vi "UpdateMovingCursor XYGraph.vi"(8 "Coords":T1, 9 "CtlRef":refnum<vi>) -> ()   [LabVIEW 2013, in "main.lvlib"]
uses:
  main.lvlib
  <vilib>/Utility/miscctls.llb/LVPoint32TypeDef.ctl
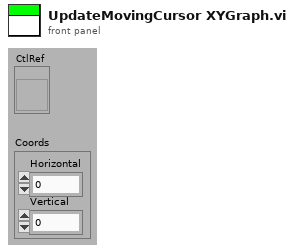
[diagram p1: front panel]
types:
  T1 = typedef "LVPoint32TypeDef.ctl" = cluster{"Horizontal":i32, "Vertical":i32}
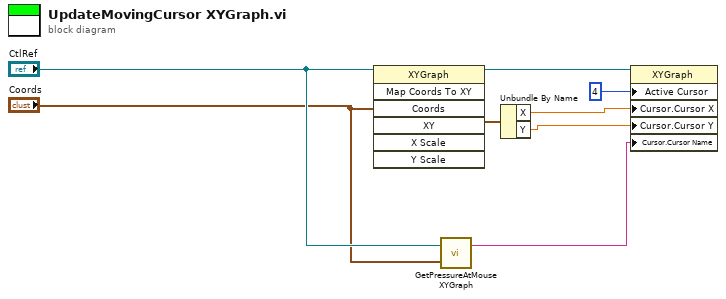
[diagram p0: block diagram]
diagram:
  n1 = invoke class="XYGraph" method="Map Coords To XY"(reference="CtlRef", "Coords"="Coords") -> (reference out=w1:refnum<vi>, "XY"=w2:cluster{"X":dbl, "Y":dbl})  [unwired: 5 in, 5 out]
  n2 = call "GetPressureAtMouse XYGraph.vi"("Coords"="Coords", "GraphRefnum"="CtlRef") -> ("String"=w5:string)  [unwired: 1 out]
  n3 = Unbundle By Name(w2) -> ("X"=w7:dbl, "Y"=w6:dbl)
  n4 = property class="XYGraph"(reference=w1, "Active Cursor"=u32 4, "Cursor.Cursor X"=w7, "Cursor.Cursor Y"=w6, "Cursor.Cursor Name"=w5) -> ()  [unwired: 1 in, 2 out]
